vi "Launch Commissioning Optimization.vi"(8 "error in":errorcluster, 11 "SCADA in":refnum<class "EMS.lvclass">) -> (0 "error out":errorcluster, 3 "SCADA out":refnum<class "EMS.lvclass">)   [LabVIEW 2018, in "EMS Core.lvlib" / "EMS.lvclass"]
uses:
  EMS.lvclass
  C:/Users/Administrator/Desktop/LabVIEW EMS/EMS Generic Actor/EMS Generic/EMS Generic.lvclass
  C:/Program Files (x86)/National Instruments/LabVIEW 2018/vi.lib/ActorFramework/Actor/Actor.lvclass
  Optimization/Commissioning Actor/Commissioning/Commissioning.lvclass
  C:/Users/Administrator/Desktop/LabVIEW EMS/Device Communication and Control Abstract Actor/Device Communication and Control Abstract/Device Communication and Control Abstract.lvclass
  EMS Messages/Activate or Blackstart Notification Msg/Activate or Blackstart Notification Msg.lvclass
  C:/Users/Administrator/Desktop/LabVIEW EMS/Optimization/Commissioning Actor/Commissioning Messages/Activate or Blackstart Msg/Activate or Blackstart Msg.lvclass
  Optimization/Commissioning Actor/Commissioning/Commissioning.lvclass/Commissioning.ctl
  EMS.lvclass/EMS.ctl
  <vilib>/ActorFramework/Actor/Actor.lvclass
  Global Variables/Global Variables.vi
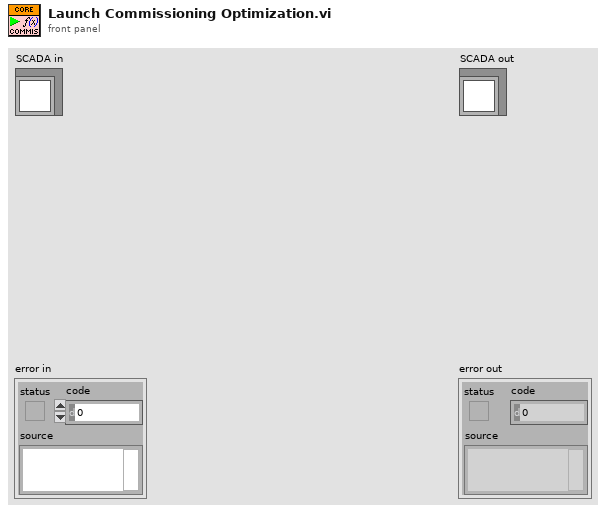
[diagram p1: front panel]
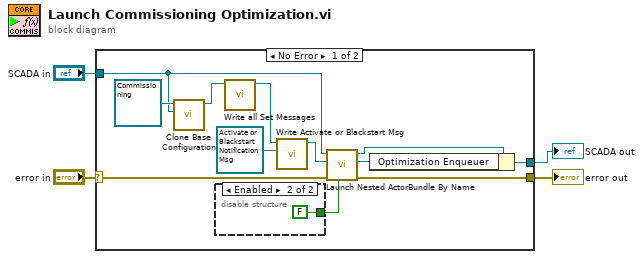
[diagram p0: block diagram]
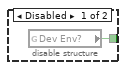
[diagram p2: hidden frame]
diagram:
  n1 = case shown="No Error" "error in" {
    selector: "error in" -> [w9 w20]
    tunnel: [w15 w20] -> w3
    tunnel: [w14 w19] -> w1
    tunnel: "SCADA in" -> [w7 w19]
    frame No Error {
      n2 = call-dynamic "Clone Base Configuration.vi"("Source Object"=w7, "Target Object in"=refnum<class "Commissioning.lvclass"> refnum ("Commissioning Actor.lvlib:Commissioning.lvclass")) -> ("Target Object out"=w6:refnum<class "Commissioning.lvclass">)  [unwired: 9 in]
      n3 = disable-structure shown="Enabled" {
        disable-tunnel: [w17 FALSE ("Open Actor Core front panel? (F)")] -> w5
        frame Disabled {
          n4 = global read "Global Variables.vi" "Dev Env?"() -> (w17:bool)
        }
        frame Enabled {
        }
      }
      n5 = call "Write all Set Messages.vi"("Device Communication and Control Abstract In"=w6) -> ("Device Communication and Control Abstract Out"=w12:refnum<class "Commissioning.lvclass">)  [unwired: 10 in]
      n6 = call "Write Activate or Blackstart Msg.vi"("Activate or Blackstart Msg"=refnum<class "Activate or Blackstart Notification Msg.lvclass"> refnum ("SCADA Core.lvlib:Activate or Blackstart Notification Msg.lvclass"), "Commissioning in"=w12) -> ("Commissioning out"=w11:refnum<class "Commissioning.lvclass">)  [unwired: 9 in]
      n7 = call <vilib>:"Launch Nested Actor.vi"("Open Actor Core front panel? (F)"=w5, "error in (no error)"=w9, "Nested Actor"=w11, "Caller Actor in"=w7) -> ("error out"=w15:errorcluster, "Nested Actor's Enqueuer"=w13:refnum<class "Message Enqueuer.lvclass">, "Caller Actor out"=w16:refnum<class "EMS.lvclass">)  [unwired: 5 in]
      n8 = Bundle By Name(cluster=w16, "Optimization Enqueuer"=w13) -> (w14:refnum<class "EMS.lvclass">)
    }
    frame Error {
    }
  }
  "error out" <- w3
  "SCADA out" <- w1
